vi "Initialise.vi"(8 "error in (no error)":errorcluster, 10 "Message in":refnum<class "InitialiseMessage.lvclass">, 11 "Retiga in":refnum<class "Retiga.lvclass">) -> (0 "error out":errorcluster, 3 "Retiga out":refnum<class "Retiga.lvclass">)   [LabVIEW 2012, in "Retiga.lvclass"]
doc: "This method is called when an initialise message is received. It mainly initialises the RabbitMQ connectivity. \n\nOverride this method when your component needs special initialisation (e.g. of software or hardware resources). In that case, don't forget to call the parent for proper implementation. If your component owns subcomponents, they count as resources, so you have to initialise them by calling their own initialise functions"
uses:
  Retiga.lvclass
  <vilib>/Distrio/Murmex/InitialiseMessage/InitialiseMessage.lvclass
  <vilib>/Distrio/Murmex/Murmex/Murmex.lvclass
  Retiga.lvclass/Retiga.ctl
panel:
  # "This method is called when the INTIALISE\ntrigger is sent. \n\nOverride this method when your component needs to\nrespond to this trigger. \n\nCall parent for proper implementation"
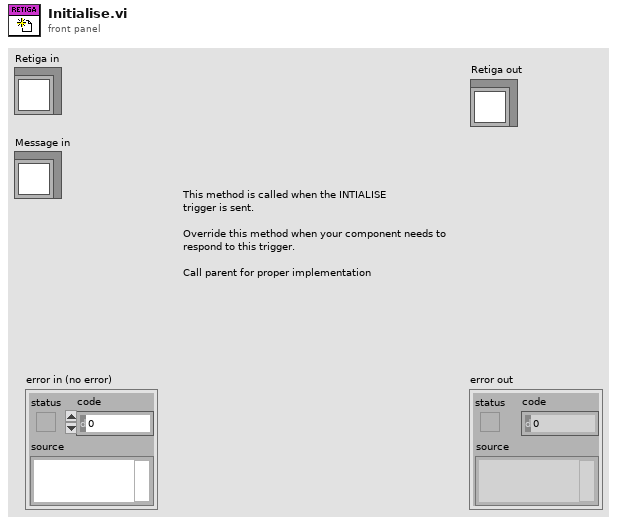
[diagram p1: front panel]
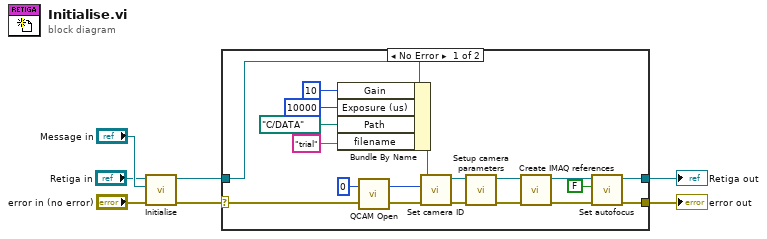
[diagram p0: block diagram]
diagram:
  n1 = call-parent "Initialise.vi"("error in (no error)"="error in (no error)", "Message in"="Message in", "Murmex in"="Retiga in") -> ("error out"=w4:errorcluster, "Murmex out"=w2:refnum<class "Retiga.lvclass">)  [unwired: 7 in]
  n2 = case shown="No Error" w4 {
    selector: w4 -> [w25 w28]
    tunnel: [w13 w28] -> w3
    tunnel: w2 -> [w24 w27]
    tunnel: [w14 w27] -> w1
    frame No Error {
      n3 = Bundle By Name(cluster=w24, "Gain"=10 ("settings.Gain"), "Exposure (us)"=10000 ("settings.Exposure (us)"), "Path"=path "C:/DATA" ("settings.Path"), "filename"="trial" ("settings.filename")) -> (w9:refnum<class "Retiga.lvclass">)
      n4 = call <userlib>:"QCAM Open.vi"("error in (no error)"=w25, "cameraId"=u32 0) -> ("error out"=w12:errorcluster, "cameraId out"=w8:u32)
      n5 = call-dynamic "Set camera ID.vi"("error in (no error)"=w12, "camera ID"=w8, "Retiga in"=w9) -> ("error out"=w11:errorcluster, "Retiga out"=w10:refnum<class "Retiga.lvclass">)  [unwired: 7 in]
      n6 = call-dynamic "Setup camera parameters.vi"("error in (no error)"=w11, "Retiga in"=w10) -> ("error out"=w23:errorcluster, "Retiga out"=w22:refnum<class "Retiga.lvclass">)  [unwired: 8 in]
      n7 = call-dynamic "Create IMAQ references.vi"("error in (no error)"=w23, "Retiga in"=w22) -> ("error out"=w21:errorcluster, "Retiga out"=w20:refnum<class "Retiga.lvclass">)  [unwired: 8 in]
      n8 = call-dynamic "Set autofocus.vi"("error in (no error)"=w21, "autofocusing?"=FALSE, "Retiga in"=w20) -> ("error out"=w13:errorcluster, "Retiga out"=w14:refnum<class "Retiga.lvclass">)  [unwired: 7 in]
    }
    frame Error {
    }
  }
  "error out" <- w3
  "Retiga out" <- w1
